vi "Take Snapshot.vi"(8 "error in (no error)":errorcluster, 11 "Snapshot Label":string) -> (0 "error out":errorcluster)   [LabVIEW 2009]
uses:
  Data Access Objects/Metadata/Persistant DAO Actions.ctl
  Apps/Yes No Button.ctl
  Archive File Type.ctl
  LogFileType.ctl
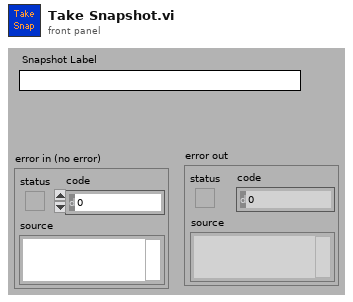
[diagram p1: front panel]
types:
  T1 = typedef "Yes No Button.ctl" = bool
  T2 = typedef "Persistant DAO Actions.ctl" = enum16{"Init", "Get", "Set", "Load", "Save"}
  T3 = typedef "Number Of LBCBs.ctl" = enum16{"1", "2"}
  T4 = typedef "App Parameters.ctl" = cluster{"Monitor Loop":T5, "Ramp Time":T5, "Log Loop":T5, "TCP to DAQ":T5, "Logging Directory":path, "Log File Size (MBytes)":i64, "Volt Logging Loop":T5, "2 LBCB Archiving Mode":bool}
  T5 = typedef "Timing Parameters.ctl" = cluster{"Interval":dbl, "Rate ":dbl}
  T6 = typedef "Dataset Transaction Id.ctl" = cluster{"Dataset Source":T7, "Dataset Type":T8, "Hold":T1, "Volts":T1, "Tag":string}
  T7 = typedef "Dataset Source.ctl" = enum16{"LBCB 1", "LBCB 2", "Combined", "External Sensors"}
  T8 = typedef "Dataset Type.ctl" = enum16{"LVDT", "Load Cell", "Actuator Command", "Servo Error", "Displacement Command", "Displacement", "Force"}
  T9 = typedef "Archive File Type.ctl" = enum16{"LBCB1", "LBCB2", "ExternalSensors", "Combined"}
  T10 = typedef "LogFileType.ctl" = enum16{"Continuous", "Step", "Volts", "Offsets", "DLL  Errors", "Snapshot", "Commands", "StiffnessUpdates", "End List"}
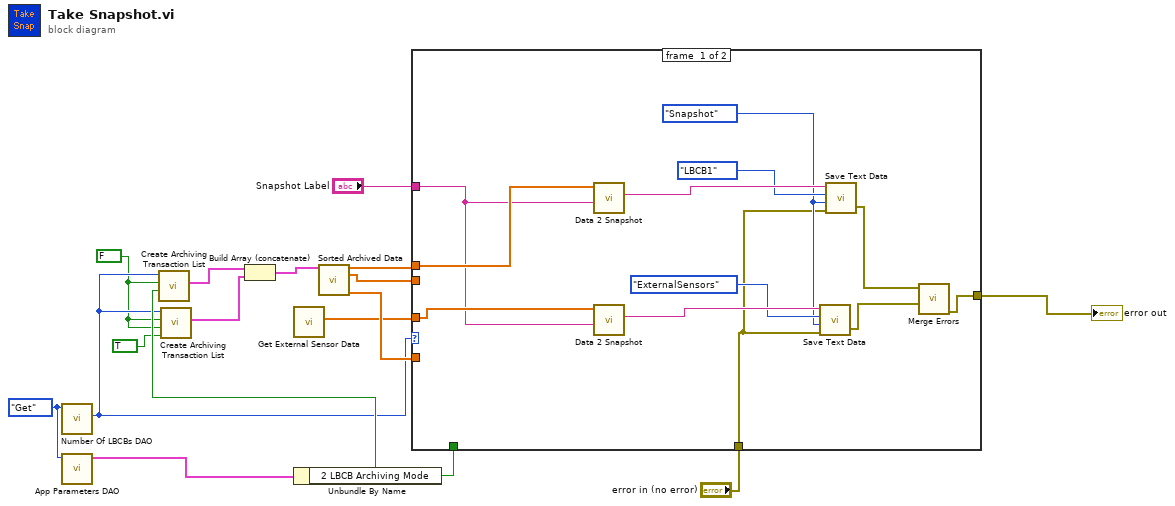
[diagram p0: block diagram]
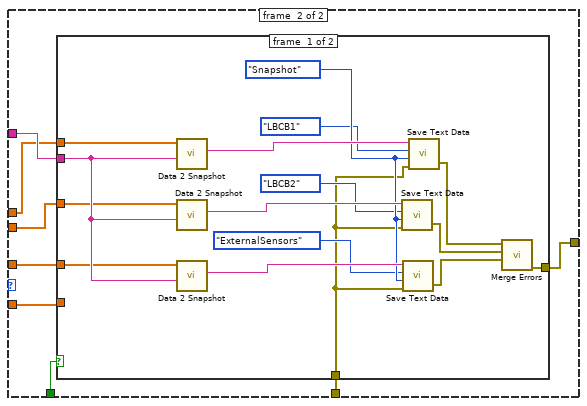
[diagram p2: hidden frame]
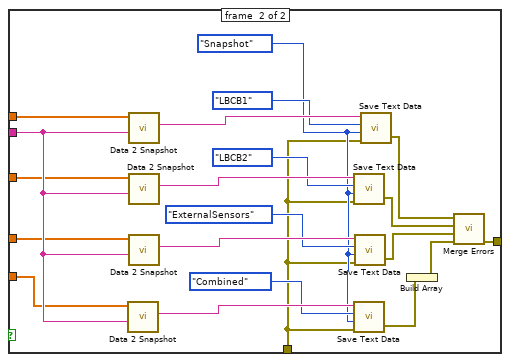
[diagram p3: hidden frame]
diagram:
  w7 = T1 FALSE ("Hold")
  w14 = Persistant_DAO_Actions."Get" ("Actions")
  n1 = call "Number Of LBCBs DAO.vi"("Actions"=w14) -> ("Number of\nLBCBs Out"=w8:T3)  [unwired: 7 in, 3 out]
  n2 = call "App Parameters DAO.vi"("Actions"=w14) -> ("Application Timing and Logging Out"=w13:T4)  [unwired: 8 in, 2 out]
  n3 = call "Create Archiving Transaction List.vi"("Volts Only"=TRUE ("Include Volts"), "Combined LBCBs"=w7, "Hold"=w7, "Number of LBCBs"=w8) -> ("Transactions"=w5:T6[])  [unwired: 7 in]
  n4 = call "Get External Sensor Data.vi"() -> ("Data Out"=w4:dbl[])  [unwired: 8 in, 3 out]
  n5 = Unbundle By Name(w13) -> ("2 LBCB Archiving Mode"=w10:bool)
  n6 = call "Create Archiving Transaction List.vi"("Combined LBCBs"=w10, "Hold"=w7, "Number of LBCBs"=w8) -> ("Transactions"=w11:T6[])  [unwired: 8 in]
  n7 = Build Array (concatenate)(w11, w5) -> (w6:T6[])
  n8 = call "Sorted Archived Data.vi"("Transactions"=w6) -> ("LBCB 1 \nwith Volts"=w3:dbl[], "LBCB 2\nwith Volts"=w2:dbl[], "Combined"=w12:dbl[])  [unwired: 10 in, 2 out]
  n9 = case shown="\"1\", Default" w8 {
    tunnel: [w18 w36] -> w16
    tunnel: "Snapshot Label" -> [w19 w35]
    tunnel: w10 -> [_ w34]
    tunnel: w3 -> [w21 w33]
    tunnel: w2 -> [_ w32]
    tunnel: w4 -> [w20 w31]
    tunnel: w12 -> [_ w30]
    tunnel: "error in (no error)" -> [w17 w29]
    frame #0 {
      w22 = LogFileType."Snapshot" ("LogFile Type")
      n10 = call "Data 2 Snapshot.vi"("Snapshot Label"=w19, "Data"=w21) -> ("Record"=w26:string)  [unwired: 9 in]
      n11 = call "Data 2 Snapshot.vi"("Snapshot Label"=w19, "Data"=w20) -> ("Record"=w25:string)  [unwired: 9 in]
      n12 = call "Save Text Data.vi"("String"=w25, "Archive File Type"=Archive_File_Type."ExternalSensors", "LogFile Type"=w22, "error in"=w17) -> ("error out"=w27:errorcluster)  [unwired: 1 in, 1 out]
      n13 = call "Save Text Data.vi"("String"=w26, "Archive File Type"=Archive_File_Type."LBCB1", "LogFile Type"=w22, "error in"=w17) -> ("error out"=w28:errorcluster)  [unwired: 1 in, 1 out]
      n14 = call <vilib>:"Merge Errors.vi"("error in 3 (no error)"=w27, "error in 1 (no error)"=w28) -> ("error out"=w18:errorcluster)  [unwired: 5 in]
    }
    frame #1 {
      n15 = case shown="False" w34 {
        tunnel: [w52 w73] -> w36
        tunnel: w35 -> [w48 w58]
        tunnel: w33 -> [w40 w57]
        tunnel: w32 -> [w39 w56]
        tunnel: w31 -> [w38 w55]
        tunnel: w30 -> [_ w54]
        tunnel: w29 -> [w37 w53]
        frame #0 {
          w44 = LogFileType."Snapshot" ("LogFile Type")
          n16 = call "Data 2 Snapshot.vi"("Snapshot Label"=w48, "Data"=w40) -> ("Record"=w47:string)  [unwired: 9 in]
          n17 = call "Data 2 Snapshot.vi"("Snapshot Label"=w48, "Data"=w39) -> ("Record"=w46:string)  [unwired: 9 in]
          n18 = call "Data 2 Snapshot.vi"("Snapshot Label"=w48, "Data"=w38) -> ("Record"=w45:string)  [unwired: 9 in]
          n19 = call "Save Text Data.vi"("String"=w46, "Archive File Type"=Archive_File_Type."LBCB2", "LogFile Type"=w44, "error in"=w37) -> ("error out"=w50:errorcluster)  [unwired: 1 in, 1 out]
          n20 = call "Save Text Data.vi"("String"=w45, "Archive File Type"=Archive_File_Type."ExternalSensors", "LogFile Type"=w44, "error in"=w37) -> ("error out"=w49:errorcluster)  [unwired: 1 in, 1 out]
          n21 = call "Save Text Data.vi"("String"=w47, "Archive File Type"=Archive_File_Type."LBCB1", "LogFile Type"=w44, "error in"=w37) -> ("error out"=w51:errorcluster)  [unwired: 1 in, 1 out]
          n22 = call <vilib>:"Merge Errors.vi"("error in 3 (no error)"=w49, "error in 2 (no error)"=w50, "error in 1 (no error)"=w51) -> ("error out"=w52:errorcluster)  [unwired: 4 in]
        }
        frame #1 {
          w61 = LogFileType."Snapshot" ("LogFile Type")
          n23 = call "Data 2 Snapshot.vi"("Snapshot Label"=w58, "Data"=w54) -> ("Record"=w63:string)  [unwired: 9 in]
          n24 = call "Data 2 Snapshot.vi"("Snapshot Label"=w58, "Data"=w57) -> ("Record"=w69:string)  [unwired: 9 in]
          n25 = call "Data 2 Snapshot.vi"("Snapshot Label"=w58, "Data"=w56) -> ("Record"=w68:string)  [unwired: 9 in]
          n26 = call "Data 2 Snapshot.vi"("Snapshot Label"=w58, "Data"=w55) -> ("Record"=w67:string)  [unwired: 9 in]
          n27 = call "Save Text Data.vi"("String"=w68, "Archive File Type"=Archive_File_Type."LBCB2", "LogFile Type"=w61, "error in"=w53) -> ("error out"=w71:errorcluster)  [unwired: 1 in, 1 out]
          n28 = call "Save Text Data.vi"("String"=w63, "Archive File Type"=Archive_File_Type."Combined", "LogFile Type"=w61, "error in"=w53) -> ("error out"=w60:errorcluster)  [unwired: 1 in, 1 out]
          n29 = call "Save Text Data.vi"("String"=w67, "Archive File Type"=Archive_File_Type."ExternalSensors", "LogFile Type"=w61, "error in"=w53) -> ("error out"=w70:errorcluster)  [unwired: 1 in, 1 out]
          n30 = call "Save Text Data.vi"("String"=w69, "Archive File Type"=Archive_File_Type."LBCB1", "LogFile Type"=w61, "error in"=w53) -> ("error out"=w72:errorcluster)  [unwired: 1 in, 1 out]
          n31 = Build Array(w60) -> (w59:errorcluster[])
          n32 = call <vilib>:"Merge Errors.vi"("error array in"=w59, "error in 3 (no error)"=w70, "error in 2 (no error)"=w71, "error in 1 (no error)"=w72) -> ("error out"=w73:errorcluster)  [unwired: 3 in]
        }
      }
    }
  }
  "error out" <- w16
